vi "S2C_STEP_UpdateSettings.vi"(8 "Error In":errorcluster, 9 "Cell Position":T1, 10 "ItemTag":string, 11 "CtlRef":refnum<vi>) -> (0 "Error Out":errorcluster)   [LabVIEW 2015]
doc: "Loads the popup menu for the selected Fornax command parameter."
uses:
  <vilib>/Utility/miscctls.llb/LVRowAndColumnTypeDef.ctl
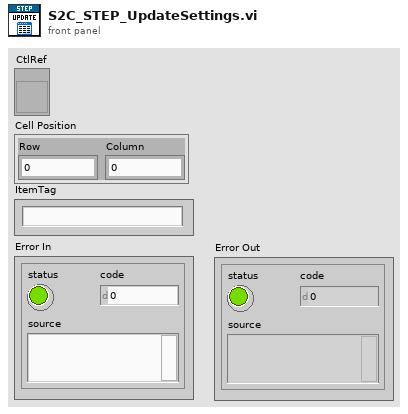
[diagram p1: front panel]
types:
  T1 = typedef "LVRowAndColumnTypeDef.ctl" = cluster{"Row":i32, "Column":i32}
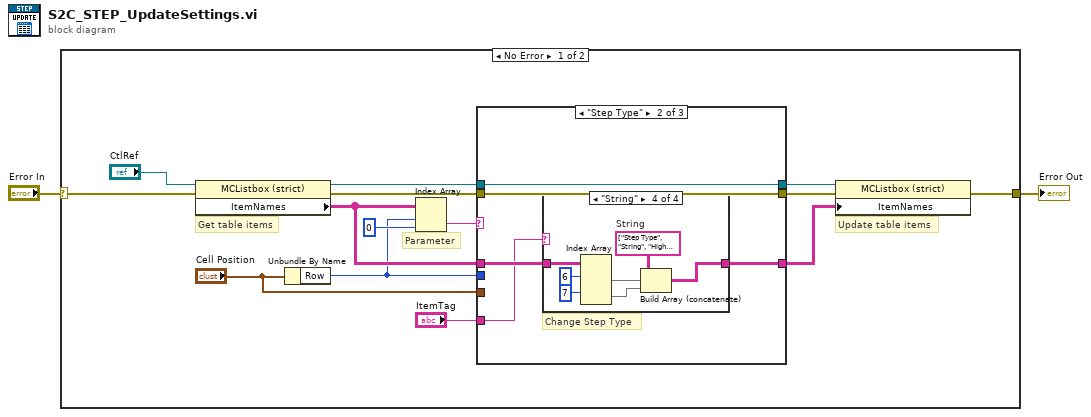
[diagram p0: block diagram]
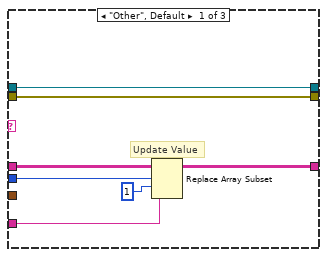
[diagram p2: hidden frame]
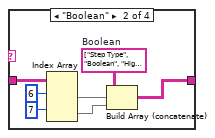
[diagram p4: hidden frame]
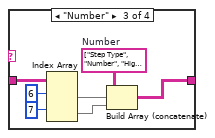
[diagram p5: hidden frame]
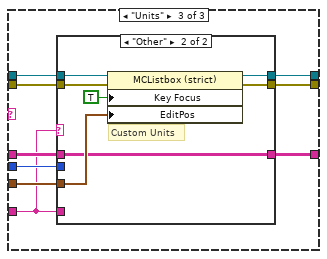
[diagram p6: hidden frame]
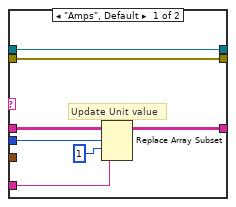
[diagram p7: hidden frame]
diagram:
  n1 = case shown="No Error" "Error In" {
    selector: "Error In" -> [w16 w74]
    tunnel: [w8 w74] -> w1
    frame No Error {
      # "Update table items"
      # "Parameter"
      # "Get table items"
      n2 = property class="MCListbox (strict)"(reference="CtlRef", error in=w16) -> (reference out=w5:refnum<vi>, error out=w11:errorcluster, "ItemNames"=w12:string[][])
      n3 = Unbundle By Name("Cell Position") -> ("Row"=w7:i32)
      n4 = Index Array(array=w12, index (row)=w7, index (col)=0 ("disabled index (col)")) -> (element=w13:string)
      n5 = case shown="\"Step Type\"" w13 {
        tunnel: w12 -> [w23 w27 w59]
        tunnel: [w21 w28 w57] -> w9
        tunnel: w11 -> [w18 w26 w52]
        tunnel: [w18 w26 w54] -> w10
        tunnel: w7 -> [w22 _ w58]
        tunnel: "ItemTag" -> [w19 w24 w51]
        tunnel: w5 -> [w17 w25 w56]
        tunnel: "Cell Position" -> [_ _ w55]
        tunnel: [w17 w25 w53] -> w3
        frame "Other", Default {
          # "Update Value"
          n6 = Replace Array Subset(array=w23, new element=w19, index (row)=w22, index (col)=1 ("disabled index (col)")) -> (w21:string[][])
        }
        frame "Step Type" {
          # "Change Step Type"
          n7 = case shown="\"String\"" w24 {
            tunnel: [w29 w32 w40 w47] -> w28
            tunnel: w27 -> [w29 w36 w43 w50]
            frame "Other", Default {
            }
            frame "Boolean" {
              w34 = string[][] [["Step Type", "Boolean"], ["High Limit", "True"], ["High Limit Comparison", "EQ"], ["Low Limit", "True"], ["Low Limit Comparison", "EQ"], ["Units", "None"]]  # Boolean
              n8 = Index Array(array=w36, index (row) #1=6 ("index (row)"), index (row) #2=7 ("index (row)")) -> (element #1=w33:string[], element #2=w31:string[])  [unwired: 2 in]
              n9 = Build Array (concatenate)(w34, w33, w31) -> (w32:string[][])
            }
            frame "Number" {
              w39 = string[][] [["Step Type", "Number"], ["High Limit", "0"], ["High Limit Comparison", "LE"], ["Low Limit", "0"], ["Low Limit Comparison", "GE"], ["Units", "None"]]  # Number
              n10 = Index Array(array=w43, index (row) #1=6 ("index (row)"), index (row) #2=7 ("index (row)")) -> (element #1=w41:string[], element #2=w37:string[])  [unwired: 2 in]
              n11 = Build Array (concatenate)(w39, w41, w37) -> (w40:string[][])
            }
            frame "String" {
              w46 = string[][] [["Step Type", "String"], ["High Limit", "Success"], ["High Limit Comparison", "EQ"], ["Low Limit", "Success"], ["Low Limit Comparison", "EQ"], ["Units", "None"]]  # String
              n12 = Index Array(array=w50, index (row) #1=6 ("index (row)"), index (row) #2=7 ("disabled index (col)")) -> (element #1=w48:string[], element #2=w44:string[])  [unwired: 2 in]
              n13 = Build Array (concatenate)(w46, w48, w44) -> (w47:string[][])
            }
          }
        }
        frame "Units" {
          n14 = case shown="\"Other\"" w51 {
            tunnel: w59 -> [w66 w70]
            tunnel: w58 -> [w65 _]
            tunnel: [w64 w70] -> w57
            tunnel: w51 -> [w62 _]
            tunnel: w56 -> [w61 w73]
            tunnel: w55 -> [_ w71]
            tunnel: [w60 w69] -> w54
            tunnel: [w61 w68] -> w53
            tunnel: w52 -> [w60 w67]
            frame "Amps", Default {
              # "Update Unit value"
              n15 = Replace Array Subset(array=w66, new element=w62, index (row)=w65, index (col)=1 ("disabled index (col)")) -> (w64:string[][])
            }
            frame "Other" {
              # "Custom Units"
              n16 = property class="MCListbox (strict)"(reference=w73, error in=w67, "Key Focus"=TRUE, "EditPos"=w71) -> (reference out=w68:refnum<vi>, error out=w69:errorcluster)
            }
          }
        }
      }
      n17 = property class="MCListbox (strict)"(reference=w3, error in=w10, "ItemNames"=w9) -> (error out=w8:errorcluster)  [unwired: 1 out]
    }
    frame Error {
    }
  }
  "Error Out" <- w1
